vi "串口接收数据.vi"(11 "VISA引用句柄输入":refnum<visa-resource-name>) -> ()   [LabVIEW 2016]
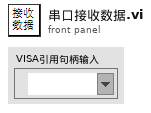
[diagram p1: front panel]
types:
  T1 = cluster{"read buffer":string, "return count":u32}
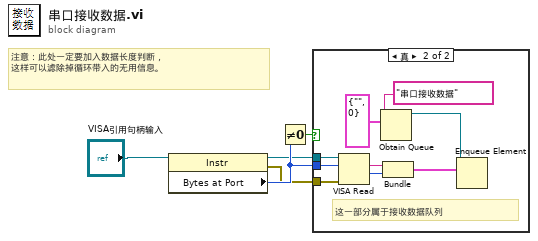
[diagram p0: block diagram]
diagram:
  # "注意：此处一定要加入数据长度判断，\n这样可以滤除掉循环带入的无用信息。"
  n1 = property class="Instr"(reference="VISA引用句柄输入") -> (reference out=w1:refnum<visa-resource-name>, error out=w2:errorcluster, "Bytes at Port"=w5:u32)  [unwired: 1 in]
  n2 = Not Equal To 0?(x=w5) -> (x != 0?=w4:bool)
  n3 = case shown="真" w4 {
    tunnel: w1 -> [_ w14]
    tunnel: w2 -> [_ w13]
    tunnel: w5 -> [_ w12]
    frame False {
    }
    frame True {
      # "这一部分属于接收数据队列"
      n4 = VISA Read(VISA resource name=w14, byte count=w12, error in (no error)=w13) -> (read buffer=w11:string, return count=w10:u32)  [unwired: 2 out]
      n5 = Obtain Queue(name (unnamed)="串口接收数据" ("名称（未命名）"), element data type=cluster{"接收字符串":string, "接收数据量":u32} {"接收字符串"="", "接收数据量"=0}) -> (queue out=w6:refnum<queue>)  [unwired: 3 in, 2 out]
      n6 = Bundle("read buffer"=w11, "return count"=w10) -> (w9:T1)  [unwired: 1 in]
      n7 = Enqueue Element(queue=w6, element=w9) -> ()  [unwired: 2 in, 3 out]
    }
  }
